vi "ttt.vi"() -> ()   [LabVIEW 2018]
uses:
  <vilib>/Platform/TimedLoop/XDataNode/timing_clust.ctl
  <vilib>/Platform/TimedLoop/XDataNode/nitl_modes.ctl
  <vilib>/Platform/TimedLoop/XDataNode/wakeup.ctl
  <vilib>/FPGAPlugInAG/myRIO-1900/niLvFpga_Open_myRIO-1900.vi
  <vilib>/rvi/interface/common/dynamic/niFpgaDynamicAddResources.vi
  <vilib>/Utility/error.llb/Error Cluster From Error Code.vi
  <vilib>/rvi/errors/niLvFpgaAdjustHostInterfaceError.vi
  <vilib>/rvi/interface/nirviOpenFPGA/nirviOpenFPGA.xnode
  FPGA Bitfiles/Dentalrobot_FPGATarget_FPGADentalroboto_PTkoih3chUc.lvbitx
  FPGA/FPGA_Dental robot output c.vi
  <vilib>/rvi/interface/nirviReadWriteControl/nirviReadWriteControl.xnode
  <vilib>/Platform/TimedLoop/XDataNode/XDataNode.xnode
  <vilib>/Platform/TimedLoop/XDataNode/XDNodeRunTimeDep.lvlib
  <vilib>/rvi/interface/Simulation/niFpgaSimulationCallBeginRW.vi
  NiFpgaLv.dll
panel:
  in  "y":dbl
  in  "OK Button":bool
  in  "DIR4":bool
  out "Position4":i32
  in  "Reset 4":bool
  in  "STBY4":bool
  in  "ENA4":bool
  in  "CH4 DC":fxp<+,32,0>
  in  "Step":u32 step=4000
  in  "Dir":bool=TRUE
  in  "stop":bool
  out "position":i32[](array[numeric])
  out "Signal":bool[](array[boolean])
  out "Finished Late?":bool
  # "Servor"
  # "Stepper"
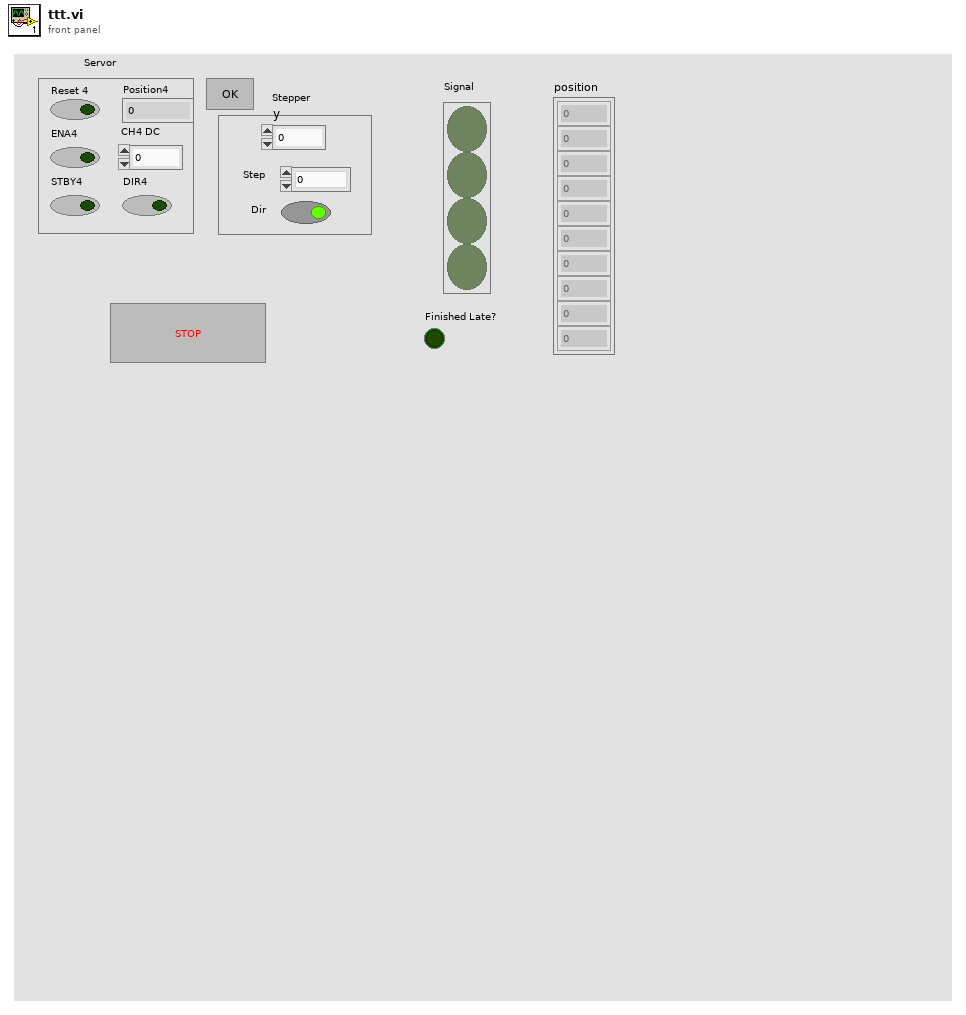
[diagram p1: front panel]
types:
  T1 = typedef "XDNodeRunTimeDep.lvlib/timing_clust.ctl" = cluster{"Expected End [f-1]":u64, "Actual End [f-1]":u64, "Finished Late? [f-1]":bool, "Expected End [i-1]":u64, "Actual End [i-1]":u64, "Finished Late? [i-1]":bool, "Expected Start [i]":u64, "Actual Start [i]":u64, "Expected Start [f]":u64, "Actual Start [f]":u64, "Source Name":string, "Structure Name":string, "Period":i64, "Deadline":i64, "Offset":i64, "Start":i64, "Priority":i32, "Timeout":i32, "Mode":T2, "Wakeup Reason":T3, "Error":errorcluster, "Source Type":string, "Secondary Source Type":string, "Global End Time":u64, "Global Start Time":u64, "Frame Duration":u64, "Iteration Duration":u64, "Assigned CPU":i32, "I/O Scan Engine Mode":u32}
  T2 = typedef "XDNodeRunTimeDep.lvlib/nitl_modes.ctl" = enum32{"No Change", "Process missed periods, maintain original phase", "Discard missed periods, maintain original phase", "Process missed periods, ignore original phase", "Discard missed periods, ignore original phase"}
  T3 = typedef "XDNodeRunTimeDep.lvlib/wakeup.ctl" = enum32{"Normal", "Aborted", "Asynchronous wakeup", "Timing source error", "Timed loop error", "Timeout"}
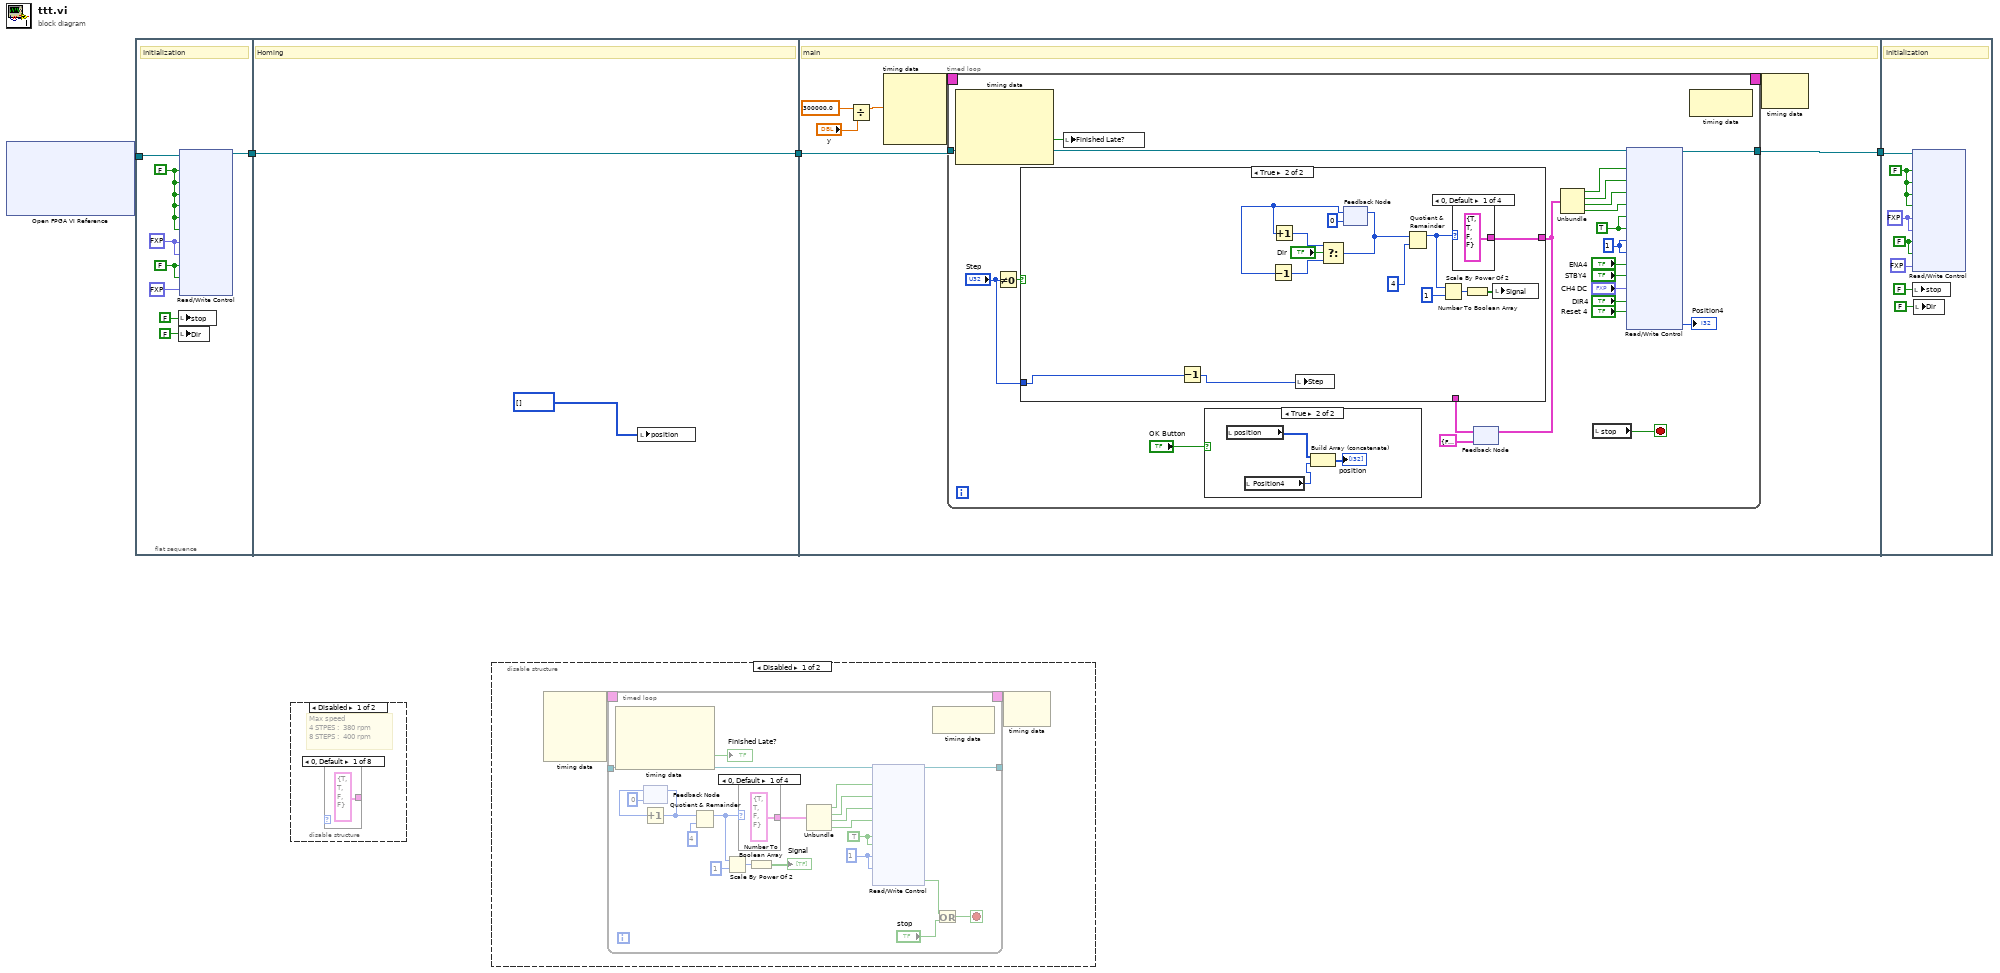
[diagram p0: block diagram]
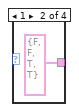
[diagram p2: hidden frame]
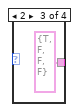
[diagram p3: hidden frame]
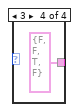
[diagram p4: hidden frame]
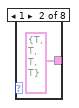
[diagram p6: hidden frame]
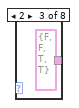
[diagram p7: hidden frame]
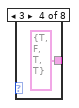
[diagram p8: hidden frame]
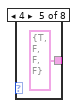
[diagram p9: hidden frame]
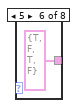
[diagram p10: hidden frame]
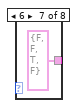
[diagram p11: hidden frame]
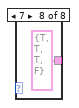
[diagram p12: hidden frame]
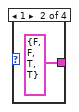
[diagram p16: hidden frame]
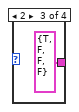
[diagram p17: hidden frame]
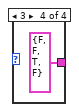
[diagram p18: hidden frame]
diagram:
  n1 = xnode "Open FPGA VI Reference"() -> ("FPGA VI Reference Out"=w3:refnum<k20>)  [unwired: 2 in, 1 out]
  n2 = flat-sequence {
    tunnel: [w11] -> w2
    tunnel: w3 -> [w9]
    tunnel: w2 -> [w14]
    tunnel: [w14] -> w1
    tunnel: [w21] -> w4
    tunnel: w1 -> [w20]
    tunnel: w4 -> [w79]
    frame #0 {
      w8 = FALSE ("ENA4")
      w10 = fxp<+,32,0> 0.0 ("CH1 DC")
      w12 = FALSE ("ENA1")
      # "Initialization"
      n3 = local write "stop"(FALSE ("stop")) -> ()
      n4 = local write "Dir"(FALSE ("Dir")) -> ()
      n5 = xnode "Read/Write Control"("FPGA VI Reference In"=w9, "ENA1"=w12, "STBY1"=w12, "DIR1"=w12, "ENA2"=w12, "STBY2"=w12, "DIR2"=w12, "CH1 DC"=w10, "CH2 DC"=w10, "ENA4"=w8, "STBY4"=w8, "CH4 DC"=fxp<+,32,0> 0.0) -> ("FPGA VI Reference Out"=w11:refnum<k20>)  [unwired: 1 in, 1 out]
    }
    frame #1 {
      # "Homing"
      n6 = local write "position"(i32[] []) -> ()
    }
    frame #2 {
      # "main"
      n7 = Divide(x=300000.0, y="y") -> (x/y=w17:dbl)
      n8 = node-c288(w17) -> (w19:T1)  [unwired: 3 in]
      n9 = timed-loop {
        timing: w19 -> [_]
        timing-out: [_] -> w18
        tunnel: [w43] -> w21
        tunnel: w20 -> [w42]
        stop <- w24 stop-if-true
        w36 = 1 ("CH1 DC")
        w40 = TRUE ("STBY1")
        n10 = node-c288() -> (w25:bool)  [unwired: 1 in, 4 out]
        n11 = Not Equal To 0?(x="Step") -> (x != 0?=w35:bool)
        n12 = local write "Finished Late?"(w25) -> ()
        n13 = case shown="True" "OK Button" {
          frame False {
          }
          frame True {
            n14 = local read "position"() -> (w46:i32[])
            n15 = local read "Position4"() -> (w45:i32)
            n16 = Build Array (concatenate)(w46, w45) -> (→"position":i32[])
          }
        }
        n17 = feedback #1(cluster{bool, bool, bool, bool} {FALSE, FALSE, FALSE, FALSE}) -> (w33:cluster{bool, bool, bool, bool})
        n18 = case shown="True" w35 {
          tunnel: [w47 w61] -> w26
          tunnel: "Step" -> [_ w54]
          tunnel: w33 -> [w47 _]
          frame False {
          }
          frame True {
            n19 = Decrement(x=w54) -> (x-1=w53:u32)
            n20 = local write "Step"(w53) -> ()
            n21 = feedback #2(0) -> (w56:i32)
            n22 = Decrement(x=w56) -> (x-1=w55:i32)
            n23 = Increment(x=w56) -> (x+1=w57:i32)
            n24 = Select(t=w57, s="Dir", f=w55) -> (s? t:f=w52:i32)
            n25 = feedback-in #2(w52) -> ()
            n26 = Quotient & Remainder(x=w52, y=4) -> (x-y*floor(x/y)=w49:i32)  [unwired: 1 out]
            n27 = Scale By Power Of 2(n=w49, x=u32 1) -> (x*2^n=w50:u32)
            n28 = case shown="0, Default" w49 {
              tunnel: [cluster{bool, bool, bool, bool} {TRUE, TRUE, FALSE, FALSE} cluster{bool, bool, bool, bool} {FALSE, FALSE, TRUE, TRUE} cluster{bool, bool, bool, bool} {TRUE, FALSE, FALSE, FALSE} cluster{bool, bool, bool, bool} {FALSE, FALSE, TRUE, FALSE}] -> w61
              frame 0, Default {
              }
              frame 1 {
              }
              frame 2 {
              }
              frame 3 {
              }
            }
            n29 = Number To Boolean Array(number=w50) -> (Boolean array=w48:bool[])
            n30 = local write "Signal"(w48) -> ()
          }
        }
        n31 = feedback-in #1(w26) -> ()
        n32 = Unbundle(w26) -> (w41:bool, w39:bool, w38:bool, w37:bool)
        n33 = local read "stop"() -> (w24:bool)
        n34 = xnode "Read/Write Control"("FPGA VI Reference In"=w42, "ENA1"=w41, "DIR1"=w39, "ENA2"=w38, "DIR2"=w37, "STBY1"=w40, "STBY2"=w40, "CH1 DC"=w36, "CH2 DC"=w36, "ENA4"="ENA4", "STBY4"="STBY4", "CH4 DC"="CH4 DC", "DIR4"="DIR4", "Reset 4"="Reset 4") -> ("FPGA VI Reference Out"=w43:refnum<k20>, "Position4"=→"Position4":i32)  [unwired: 1 in, 1 out]
        n35 = node-c288() -> ()  [unwired: 1 in, 1 out]
      }
      n36 = node-c288(w18) -> ()  [unwired: 1 out]
    }
    frame #3 {
      w76 = FALSE ("ENA4")
      w77 = fxp<+,32,0> 0.0 ("CH1 DC")
      w78 = FALSE ("ENA1")
      # "Initialization"
      n37 = xnode "Read/Write Control"("FPGA VI Reference In"=w79, "ENA1"=w78, "STBY1"=w78, "ENA2"=w78, "STBY2"=w78, "CH1 DC"=w77, "CH2 DC"=w77, "ENA4"=w76, "STBY4"=w76, "CH4 DC"=fxp<+,32,0> 0.0) -> ()  [unwired: 1 in, 2 out]
      n38 = local write "stop"(FALSE ("stop")) -> ()
      n39 = local write "Dir"(FALSE ("Dir")) -> ()
    }
  }
  n40 = disable-structure shown="Disabled" {
    frame Disabled {
      # "Max speed\n4 STPES :  380 rpm\n8 STEPS :  400 rpm"
      n41 = case shown="0, Default" {
        selector: _ -> [_ _ w83 _ _ _ _ _]
        tunnel: [cluster{bool, bool, bool, bool} {TRUE, TRUE, FALSE, FALSE} cluster{bool, bool, bool, bool} {TRUE, TRUE, TRUE, TRUE} cluster{bool, bool, bool, bool} {FALSE, FALSE, TRUE, TRUE} cluster{bool, bool, bool, bool} {TRUE, FALSE, TRUE, TRUE} cluster{bool, bool, bool, bool} {TRUE, FALSE, FALSE, FALSE} cluster{bool, bool, bool, bool} {TRUE, FALSE, TRUE, FALSE} cluster{bool, bool, bool, bool} {FALSE, FALSE, TRUE, FALSE} cluster{bool, bool, bool, bool} {TRUE, TRUE, TRUE, FALSE}] -> _
        frame 0, Default {
        }
        frame 1 {
        }
        frame 2 {
        }
        frame 3 {
        }
        frame 4 {
        }
        frame 5 {
        }
        frame 6 {
        }
        frame 7 {
        }
      }
    }
    frame Enabled {
    }
  }
  n42 = disable-structure shown="Disabled" {
    frame Disabled {
      n43 = node-c288() -> (w92:T1)  [unwired: 4 in]
      n44 = timed-loop {
        timing: w92 -> [_]
        timing-out: [_] -> w91
        tunnel: [w99] -> w90
        tunnel: [w98] -> w89
        stop <- w97 stop-if-true
        w112 = 1 ("CH1 DC")
        w113 = TRUE ("STBY1")
        n45 = node-c288() -> (→"Finished Late?":bool)  [unwired: 1 in, 3 out]
        n46 = feedback #3(0) -> (w109:i32)
        n47 = Increment(x=w109) -> (x+1=w101:i32)
        n48 = feedback-in #3(w101) -> ()
        n49 = Quotient & Remainder(x=w101, y=4) -> (x-y*floor(x/y)=w95:i32)  [unwired: 1 out]
        n50 = Scale By Power Of 2(n=w95, x=u32 1) -> (x*2^n=w107:u32)
        n51 = case shown="0, Default" w95 {
          tunnel: [cluster{bool, bool, bool, bool} {TRUE, TRUE, FALSE, FALSE} cluster{bool, bool, bool, bool} {FALSE, FALSE, TRUE, TRUE} cluster{bool, bool, bool, bool} {TRUE, FALSE, FALSE, FALSE} cluster{bool, bool, bool, bool} {FALSE, FALSE, TRUE, FALSE}] -> w106
          frame 0, Default {
          }
          frame 1 {
          }
          frame 2 {
          }
          frame 3 {
          }
        }
        n52 = Number To Boolean Array(number=w107) -> (Boolean array=→"Signal":bool[])
        n53 = Unbundle(w106) -> (w105:bool, w104:bool, w103:bool, w102:bool)
        n54 = xnode "Read/Write Control"("FPGA VI Reference In"=w99, "ENA1"=w105, "DIR1"=w104, "ENA2"=w103, "DIR2"=w102, "STBY1"=w113, "STBY2"=w113, "CH1 DC"=w112, "CH2 DC"=w112) -> ("FPGA VI Reference Out"=w98:refnum<k20>, "C1"=w93:bool)  [unwired: 1 in, 1 out]
        n55 = node-c288() -> ()  [unwired: 1 in, 1 out]
        n56 = Or(x=w93, y="stop") -> (x .or. y?=w97:bool)
      }
      n57 = node-c288(w91) -> ()  [unwired: 1 out]
    }
    frame Enabled {
    }
  }
